vi "Get Cached Elements.vi"(8 "error in":errorcluster, 10 "Index":i32, 11 "ParseGDSII in":refnum<class "ParseGDSII.lvclass">) -> (0 "error out":errorcluster, 2 "Elements":refnum<class "Geometric.lvclass">[](array[class]), 3 "ParseGDSII out":refnum<class "ParseGDSII.lvclass">)   [LabVIEW 2019, in "ParseGDSII.lvclass"]
uses:
  ParseGDSII.lvclass
  Structures/Structure.lvclass
  Elements/Geometric.lvclass
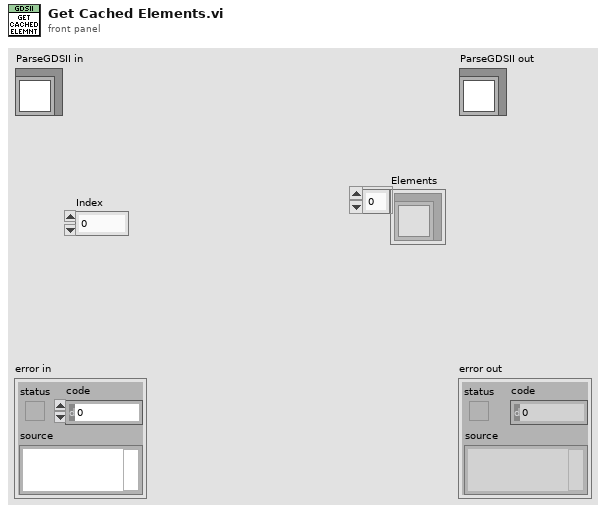
[diagram p1: front panel]
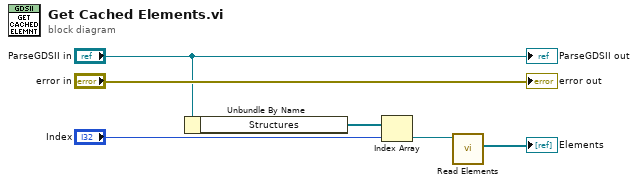
[diagram p0: block diagram]
diagram:
  n1 = Unbundle By Name("ParseGDSII in") -> ("Structures"=w5:refnum<class "Structure.lvclass">[])
  n2 = Index Array(array=w5, index="Index") -> (element=w3:refnum<class "Structure.lvclass">)
  n3 = call "Read Elements.vi"("Structure in"=w3) -> ("Elements"=→"Elements":refnum<class "Geometric.lvclass">[])  [unwired: 8 in, 2 out]
  "error out" <- "error in"
  "ParseGDSII out" <- "ParseGDSII in"
